vi "Write Default to File.vi"(8 "error in (no error)":errorcluster, 9 "Name":string, 10 "Path":path, 11 "Path Settings in":refnum<class "Path Settings.lvclass">) -> (0 "error out":errorcluster, 3 "Path Settings out":refnum<class "Path Settings.lvclass">)   [LabVIEW 2019, in "Path Settings.lvclass"]
uses:
  Path Settings.lvclass
  ObjectSettings/ObjectSettings.lvclass
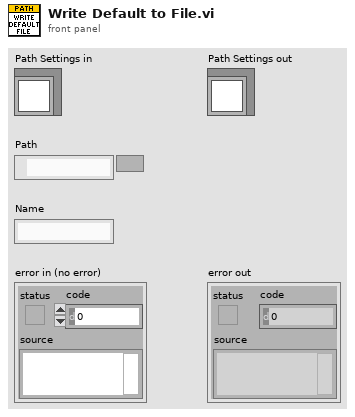
[diagram p1: front panel]
types:
  T1 = typedef "Path Settings.lvclass/Default Path Cluster.ctl" = cluster{"Fill Orientation":u16, "Smooth Segments":dbl, "Fill Spacing":dbl, "Interpolation":dbl, "Deviate":bool, "Deviation Function":cluster{"Key":string, "Value":string}}
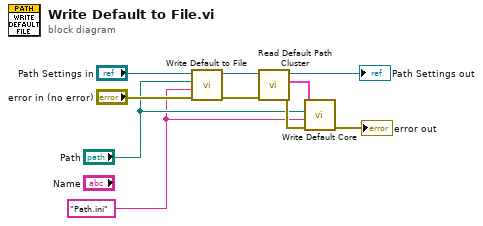
[diagram p0: block diagram]
diagram:
  w2 = "Path.ini"
  n1 = call-parent "Write Default to File.vi"("error in (no error)"="error in (no error)", "Name"=w2, "Path"="Path", "ObjectSettings in"="Path Settings in") -> ("error out"=w6:errorcluster, "ObjectSettings out"=w8:refnum<class "Path Settings.lvclass">)  [unwired: 6 in]
  n2 = call "Read Default Path Cluster.vi"("error in (no error)"=w6, "Path Settings in"=w8) -> ("error out"=w5:errorcluster, "Default Path"=w4:T1, "Path Settings out"=→"Path Settings out":refnum<class "Path Settings.lvclass">)  [unwired: 7 in]
  n3 = call "Write Default Core.vi"("error in (no error)"=w5, "Name"=w2, "Path"="Path", "Cluster In"=w4) -> ("error out"=→"error out":errorcluster)  [unwired: 6 in, 1 out]
